vi "SetTime.vi"(7 "LWSR":refnum<class "Web Request.lvclass">, 11 "time":dbl) -> ()   [LabVIEW 2014]
uses:
  <vilib>/wsapi/Web Request.lvclass
  <vilib>/nisyscfg/nisyscfg.lvlib
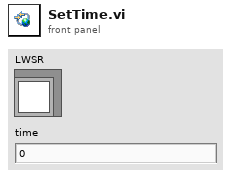
[diagram p1: front panel]
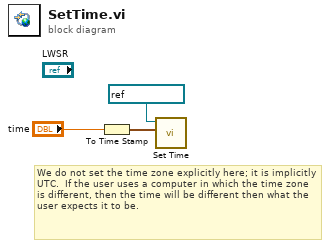
[diagram p0: block diagram]
diagram:
  # "We do not set the time zone explicitly here; it is implicitly UTC.  If the user uses a computer in which the time zone is different, then the time will be different then what the user expects it to be."
  n1 = To Time Stamp(1:"time") -> (0:w1:timestamp)
  n2 = call <vilib>:"Set Time.vi"("Time"=w1, "Session in (localhost)"=refnum<k21> "localhost") -> ()  [unwired: 6 in, 4 out]
